vi "sequence re-order.vi"(1 "seq in":string[][](array[string])) -> (0 "seq out":string[][](array[string]))   [LabVIEW 2020]
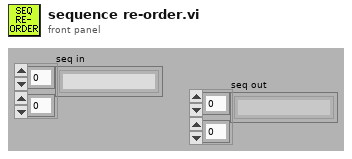
[diagram p1: front panel]
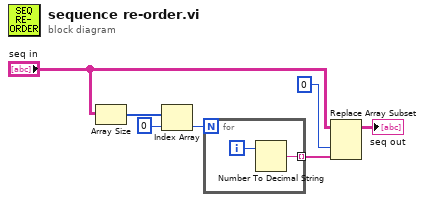
[diagram p0: block diagram]
diagram:
  n1 = Array Size(array="seq in") -> (size(s)=w5:i32[])
  n2 = Index Array(array=w5, index=0 ("disabled index (col)")) -> (element=w2:i32)
  n3 = for {
    N: w2 -> [_]
    tunnel: [w8] -> w7 mode=indexing
    i -> [w9]
    n4 = Number To Decimal String(number=w9) -> (decimal integer string=w8:string)  [unwired: 1 in]
  }
  n5 = Replace Array Subset(array="seq in", new element=w7, index (col)=0 ("disabled index (col)")) -> (→"seq out":string[][])  [unwired: 1 in]
